vi "Read Value.vi"(8 "error in (no error)":errorcluster, 11 "fixed64 in":refnum<class "fixed64.lvclass">) -> (0 "error out":errorcluster, 2 "Value":u64, 3 "fixed64 out":refnum<class "fixed64.lvclass">)   [LabVIEW 2020, in "Protobuf RAW.lvlib" / "fixed64.lvclass"]
uses:
  fixed64.lvclass
  fixed64.lvclass/fixed64.ctl
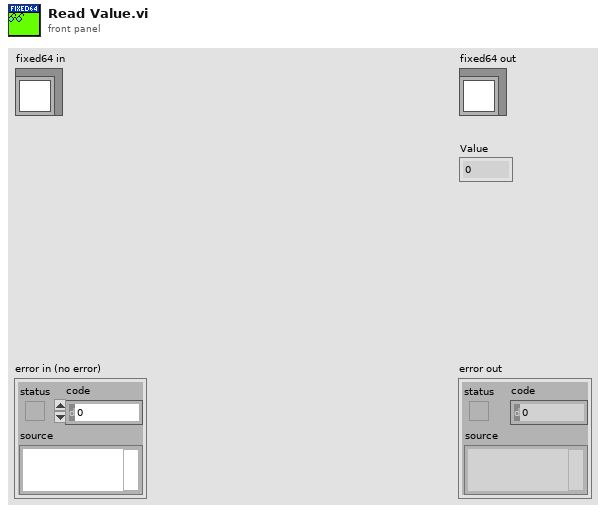
[diagram p1: front panel]
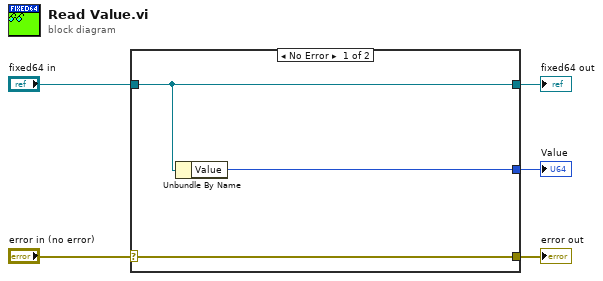
[diagram p0: block diagram]
diagram:
  n1 = case shown="No Error" "error in (no error)" {
    selector: "error in (no error)" -> [w8 w9]
    tunnel: [w8 w9] -> w4
    tunnel: [w7 w10] -> w2
    tunnel: "fixed64 in" -> [w7 w10]
    tunnel: [w6 _] -> w1
    frame No Error {
      n2 = Unbundle By Name(w7) -> ("Value"=w6:u64)
    }
    frame Error {
    }
  }
  "error out" <- w4
  "fixed64 out" <- w2
  "Value" <- w1
